vi "Get Cross Sectional Ext Area.vi"(10 "l (nm)":dbl) -> (2 "CAext (m2)":dbl)   [LabVIEW 2016, in "Atmospheric Library.lvlib"]
uses:
  Atmospheric Library.lvlib
  Gas.ctl
  Atmospheric Constants.vi
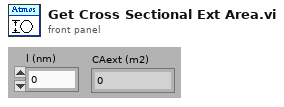
[diagram p1: front panel]
types:
  T1 = typedef "Atmospheric Library.lvlib/Gas.ctl" = enum16{"Air"}
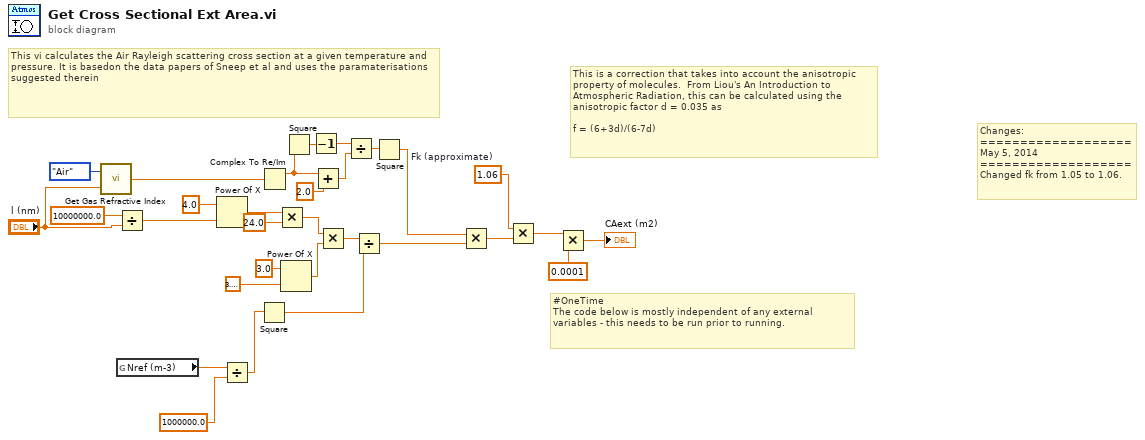
[diagram p0: block diagram]
diagram:
  w1 = 1.06  # Fk (approximate)
  # "Changes:\n===================\nMay 5, 2014\n===================\nChanged fk from 1.05 to 1.06."
  # "This is a correction that takes into account the anisotropic property of molecules.  From Liou's An Introduction to Atmospheric Radiation, this can be calculated using the anisotropic factor d = 0.035 as \n\nf = (6+3d)/(6-7d)"
  # "#OneTime\nThe code below is mostly independent of any external variables - this needs to be run prior to running."
  # "This vi calculates the Air Rayleigh scattering cross section at a given temperature and pressure. It is basedon the data papers of Sneep et al and uses the paramaterisations  suggested therein"
  n1 = call "Get Gas Refractive Index.vi"("l (nm)"="l (nm)", "Gas"=Gas."Air") -> ("n"=w26:cdb)
  n2 = Divide(x=10000000.0, y="l (nm)") -> (x/y=w19:dbl)
  n3 = global read "Atmospheric Constants.vi" "Nref (m-3)"() -> (w13:dbl)
  n4 = Power Of X(1:w19, 2:4.0 ("y")) -> (0:w6:dbl)
  n5 = Divide(x=w13, y=1000000.0) -> (x/y=w11:dbl)
  n6 = Square(x=w11) -> (x^2=w3:dbl)
  n7 = Complex To Re/Im(x + iy=w26) -> (x=w25:dbl)  [unwired: 1 out]
  n8 = Multiply(x=w6, y=24.0) -> (x*y=w17:dbl)
  n9 = Power Of X(1:3.141592653589793, 2:3.0 ("y")) -> (0:w2:dbl)
  n10 = Square(x=w25) -> (x^2=w24:dbl)
  n11 = Decrement(x=w24) -> (x-1=w5:dbl)
  n12 = Add(x=w25, y=2.0) -> (x+y=w22:dbl)
  n13 = Multiply(x=w17, y=w2) -> (x*y=w14:dbl)
  n14 = Divide(x=w5, y=w22) -> (x/y=w21:dbl)
  n15 = Divide ("Cross Sectional Area")(x=w14, y=w3) -> (x/y=w28:dbl)
  n16 = Square(x=w21) -> (x^2=w20:dbl)
  n17 = Multiply(x=w20, y=w28) -> (x*y=w29:dbl)
  n18 = Multiply ("Cross Sectional Area")(x=w1, y=w29) -> (x*y=w10:dbl)
  n19 = Multiply(x=w10, y=0.0001) -> (x*y=→"CAext (m2)":dbl)
